vi "CallDeviceSubVi.vi"(4 "device conneced":bool, 6 "error in":errorcluster, 8 "State Queue":string, 9 "Data cluster":T1) -> (0 "error out":errorcluster, 1 "states out":string, 3 "Data cluster out":T1)   [LabVIEW 2013]
uses:
  dataCluster.ctl
  <vilib>/vision/Image Controls.llb/IMAQ Image.ctl
  DataQueueTypeDef.ctl
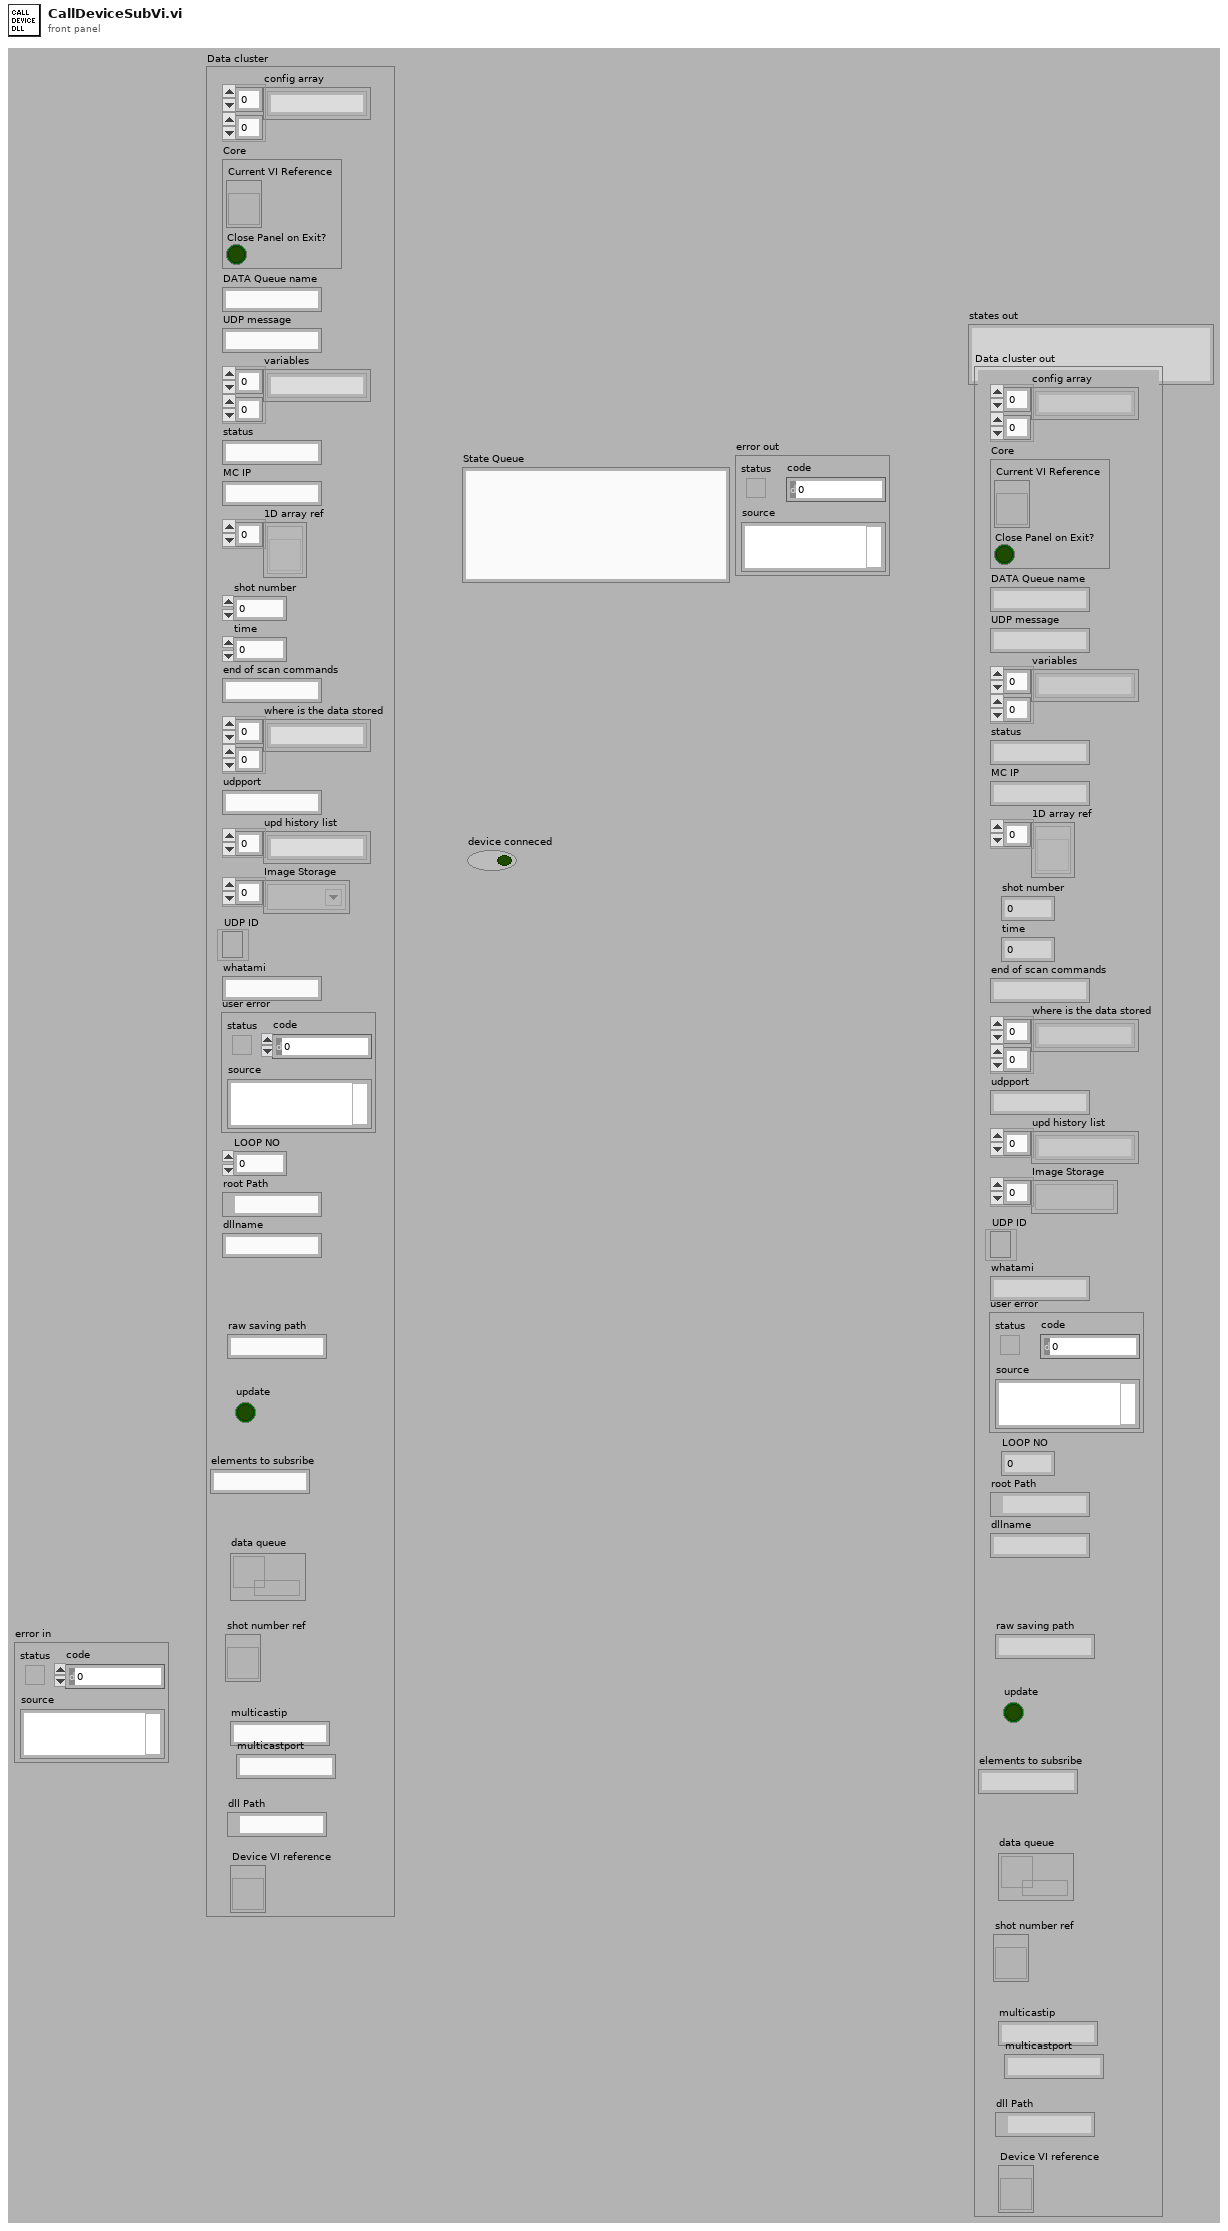
[diagram p1: front panel]
types:
  T1 = typedef "dataCluster.ctl" = cluster{"config array":string[][], "Core":cluster{"Current VI Reference":refnum<vi>, "Close Panel on Exit?":bool}, "DATA Queue name":string, "UDP message":string, "variables":string[][], "status":string, "MC IP":string, "1D array ref":refnum<vi>[], "shot number":i32, "time":u32, "end of scan commands":string, "where is the data stored":string[][], "udpport":string, "upd history list":string[], "Image Storage":T2[], "UDP ID":refnum<k16>, "whatami":string, "user error":errorcluster, "LOOP NO":u32, "root Path":path, "dllname":string, "raw saving path":string, "update":bool, "elements to subsribe":string, "data queue":refnum<queue>, "shot number ref":refnum<vi>, "multicastip":string, "multicastport":string, "dll Path":path, "Device VI reference":refnum<vi>}
  T2 = typedef "IMAQ Image.ctl" = refnum<image>
  T3 = cluster{"config array":string[][], "where is the data stored":string[][], "variables":string[][], "1D array ref":refnum<vi>[], "Image Storage":string[], "Settings":string[][]}
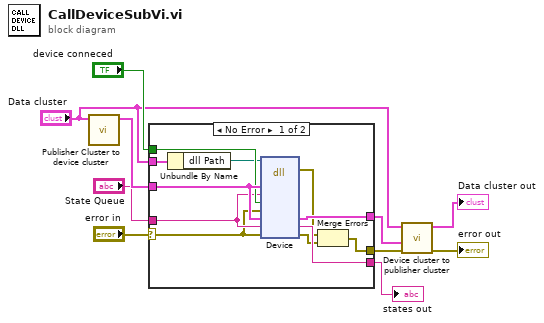
[diagram p0: block diagram]
diagram:
  n1 = call "Publisher Cluster to device cluster.vi"("publisher cluster"="Data cluster") -> ("Device cluster"=w9:T3)  [unwired: 10 in]
  n2 = case shown="No Error" "error in" {
    selector: "error in" -> [w13 w22]
    tunnel: [w14 w22] -> w6
    tunnel: [w21 w23] -> w10
    tunnel: w9 -> [w20 w24]
    tunnel: [w19 w24] -> w4
    tunnel: "device conneced" -> [w18 _]
    tunnel: "State Queue" -> [w17 w23]
    tunnel: "Data cluster" -> [w12 _]
    frame No Error {
      n3 = Unbundle By Name(w12) -> ("dll Path"=w11:path)
      n4 = dll-call lib="X:/Software/LOASIS Control System/Developers Version/Device Driver/Analysis/data/Analysis.dll" fn="Device"(path in=w11, "DeviceCluster"=w20, "State Queue"=w17, "device connected"=w18, "Error in"=w13, "DeviceClusterOut"=w20, "states out"=w17, "error out"=w13) -> (error out=w16:errorcluster, "DeviceClusterOut"=w19:T3, "states out"=w21:string, "error out"=w15:errorcluster)  [unwired: 7 in, 1 out]
      n5 = Merge Errors(w16, w15) -> (w14:errorcluster)
    }
    frame Error {
    }
  }
  "states out" <- w10
  n6 = call "Device cluster to publisher cluster.vi"("error in"=w6, "Device cluster from subVi/Dll"=w4, "old Data cluster"="Data cluster") -> ("errorout"=→"error out":errorcluster, "Data cluster out"=→"Data cluster out":T1)  [unwired: 7 in]
